vi "Close Connection Factory Session.vi"(8 "error in (no error)":errorcluster, 11 "Connection Factory Session In":refnum<data-value>) -> (0 "error out":errorcluster)   [LabVIEW 2019, in "ConnectionFactorySession.lvlib" / "ConnectionFactorySession.lvclass"]
uses:
  <vilib>/gpm_packages/@cs/Network-interface/Source/Connection Factory Session/ConnectionFactorySession/ConnectionFactorySession.lvclass
  <vilib>/gpm_packages/@cs/Network-interface/Source/Connection Factory Session/ConnectionFactorySession/ConnectionFactorySession.lvclass/ConnectionFactorySession.ctl
  <vilib>/ActorFramework/Message Enqueuer/Message Enqueuer.lvclass/Message Enqueuer.ctl
  <vilib>/ActorFramework/Message Enqueuer/Enqueue.vi
  <vilib>/ActorFramework/Stop Msg/Stop Msg.lvclass
  C:/Program Files/National Instruments/LabVIEW 2019/vi.lib/ActorFramework/Message/Message.lvclass
  <vilib>/ActorFramework/Message Priority Queue/Priority Enqueue.vi
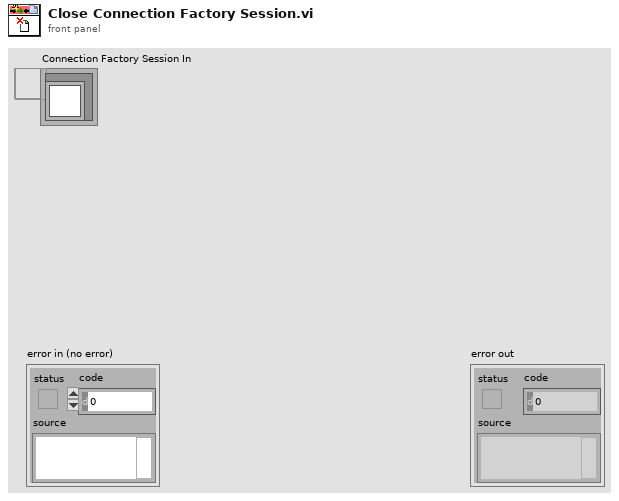
[diagram p1: front panel]
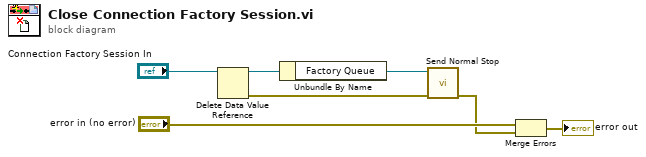
[diagram p0: block diagram]
diagram:
  n1 = Delete Data Value Reference(data value reference="Connection Factory Session In") -> (data value=w6:refnum<class "ConnectionFactorySession.lvclass">, error out=w5:errorcluster)  [unwired: 1 in]
  n2 = Unbundle By Name(w6) -> ("Factory Queue"=w4:refnum<class "Message Enqueuer.lvclass">)
  n3 = call <vilib>:"Send Normal Stop.vi"("error in (no error)"=w5, "Message Enqueuer"=w4) -> ("error out"=w2:errorcluster)  [unwired: 9 in]
  n4 = Merge Errors("error in (no error)", w2) -> (→"error out":errorcluster)
